vi "CRYGet Curve & Sensitiviy.vi"(9 "Calibration Cluster":T1={"Calibration"={"Calibration Step Name"="", "Device"="", "Correction Curve Name"="", "Equalization Curve Name"="", "Sensitivity Curve Name"="", "Corr Folder and File"="", "EQ Folder and File"="", "Sens Folder and File"="", "Corr Step size"=0, "EQ Step size"=0, "Input"=FALSE, "Last Cal Date (sec)"=timestamp(0 s since 1904-01-01), "Cha Name"="", "Corr Curve Found"=FALSE, "EQ Curve Found"=FALSE, "Sens Curve Found"=FALSE, "Signal Type"="", "Calibrated Device"="", "Hz"=0}, "Corr Curve"={"Name"="", "Curve"=[], "X data"=1, "Y data"=1, "Z data"=1, "X axis"=0, "Y axis"=1, "Z axis"=1, "X unit"="Hz", "Y unit"="", "Z unit"="deg.", "X dB ref"=1.0, "Y dB ref"=1.0, "Z dB ref"=1.0, "single val"=FALSE, "protected"=FALSE, "display X"=TRUE, "display Y"=TRUE, "display Z"=TRUE, "Test Info"="", "Step No."=0, "Plot Settings"={"Color"=0, "Interpolation"=0, "Point Style"=0, "Line Style"=0, "Point Color"=0, "Line Width"=0, "Bar Plot Style"=0, "Fill To"=0}, "AutoProtect"=FALSE}, "EQ Curve"={"Name"="", "Curve"=[], "X data"=1, "Y data"=1, "Z data"=1, "X axis"=0, "Y axis"=1, "Z axis"=1, "X unit"="Hz", "Y unit"="", "Z unit"="deg.", "X dB ref"=1.0, "Y dB ref"=1.0, "Z dB ref"=1.0, "single val"=FALSE, "protected"=FALSE, "display X"=TRUE, "display Y"=TRUE, "display Z"=TRUE, "Test Info"="", "Step No."=0, "Plot Settings"={"Color"=0, "Interpolation"=0, "Point Style"=0, "Line Style"=0, "Point Color"=0, "Line Width"=0, "Bar Plot Style"=0, "Fill To"=0}, "AutoProtect"=FALSE}, "Sens Curve"={"Name"="", "Curve"=[], "X data"=1, "Y data"=1, "Z data"=1, "X axis"=0, "Y axis"=1, "Z axis"=1, "X unit"="Hz", "Y unit"="", "Z unit"="deg.", "X dB ref"=1.0, "Y dB ref"=1.0, "Z dB ref"=1.0, "single val"=FALSE, "protected"=FALSE, "display X"=TRUE, "display Y"=TRUE, "display Z"=TRUE, "Test Info"="", "Step No."=0, "Plot Settings"={"Color"=0, "Interpolation"=0, "Point Style"=0, "Line Style"=0, "Point Color"=0, "Line Width"=0, "Bar Plot Style"=0, "Fill To"=0}, "AutoProtect"=FALSE}} {"Sens Curve"."Z data" items=["dB", "Lin"]; "Sens Curve"."X data" items=["dB", "Lin"]; "Sens Curve"."Y data" items=["dB", "Lin"]; "Sens Curve"."Z dB ref" format="%.1f"; "Sens Curve"."Z axis" items=["Log", "Lin"]; "Sens Curve"."X dB ref" format="%.1f"; "Sens Curve"."X axis" items=["Log", "Lin"]; "Sens Curve"."Y axis" items=["Log", "Lin"]; "Sens Curve"."Y dB ref" format="%.1f"; "Sens Curve"."Curve"."z" format="%.2f"; "Sens Curve"."Curve"."y" format="%.2f"; "Sens Curve"."Curve"."x" format="%.2f"; "EQ Curve"."Z data" items=["dB", "Lin"]; "EQ Curve"."X data" items=["dB", "Lin"]; "EQ Curve"."Y data" items=["dB", "Lin"]; "EQ Curve"."Z dB ref" format="%.1f"; "EQ Curve"."Z axis" items=["Log", "Lin"]; "EQ Curve"."X dB ref" format="%.1f"; "EQ Curve"."X axis" items=["Log", "Lin"]; "EQ Curve"."Y axis" items=["Log", "Lin"]; "EQ Curve"."Y dB ref" format="%.1f"; "EQ Curve"."Curve"."z" format="%.2f"; "EQ Curve"."Curve"."y" format="%.2f"; "EQ Curve"."Curve"."x" format="%.2f"; "Corr Curve"."Z data" items=["dB", "Lin"]; "Corr Curve"."X data" items=["dB", "Lin"]; "Corr Curve"."Y data" items=["dB", "Lin"]; "Corr Curve"."Z dB ref" format="%.1f"; "Corr Curve"."Z axis" items=["Log", "Lin"]; "Corr Curve"."X dB ref" format="%.1f"; "Corr Curve"."X axis" items=["Log", "Lin"]; "Corr Curve"."Y axis" items=["Log", "Lin"]; "Corr Curve"."Y dB ref" format="%.1f"; "Corr Curve"."Curve"."z" format="%.2f"; "Corr Curve"."Curve"."y" format="%.2f"; "Corr Curve"."Curve"."x" format="%.2f"; "Calibration"."EQ Step size" items=["R10", "R20", "R40", "R80", "User"]; "Calibration"."Corr Step size" items=["R10", "R20", "R40", "R80", "User"]}, 10 "Finished test? (T)":bool=TRUE, 11 "Data stack out":T4 {"Z data" items=["dB", "Lin"]; "X data" items=["dB", "Lin"]; "Y data" items=["dB", "Lin"]; "Z dB ref" format="%.1f"; "Z axis" items=["Log", "Lin"]; "X dB ref" format="%.1f"; "X axis" items=["Log", "Lin"]; "Y axis" items=["Log", "Lin"]; "Y dB ref" format="%.1f"; "Curve"."z" format="%.2f"; "Curve"."y" format="%.2f"; "Curve"."x" format="%.2f"}) -> (0 "Success?":bool, 1 "Sensitivity":dbl format="%.2f", 2 "corr-out curve":cluster{"x":dbl, "y":dbl, "z":dbl}[](array[cluster]) {"z" format="%.2f"; "y" format="%.2f"; "x" format="%.2f"}, 3 "eq- out curve":cluster{"x":dbl, "y":dbl, "z":dbl}[](array[cluster]) {"z" format="%.2f"; "y" format="%.2f"; "x" format="%.2f"})   [LabVIEW 2013]
uses:
  Typedef Control/CRYData Cluster Array.ctl
  Typedef Control/CRYData Cluster.ctl
  Typedef Control/CRYCalibration 2DCluster.ctl
  Typedef Control/CRYCalibration Cluster.ctl
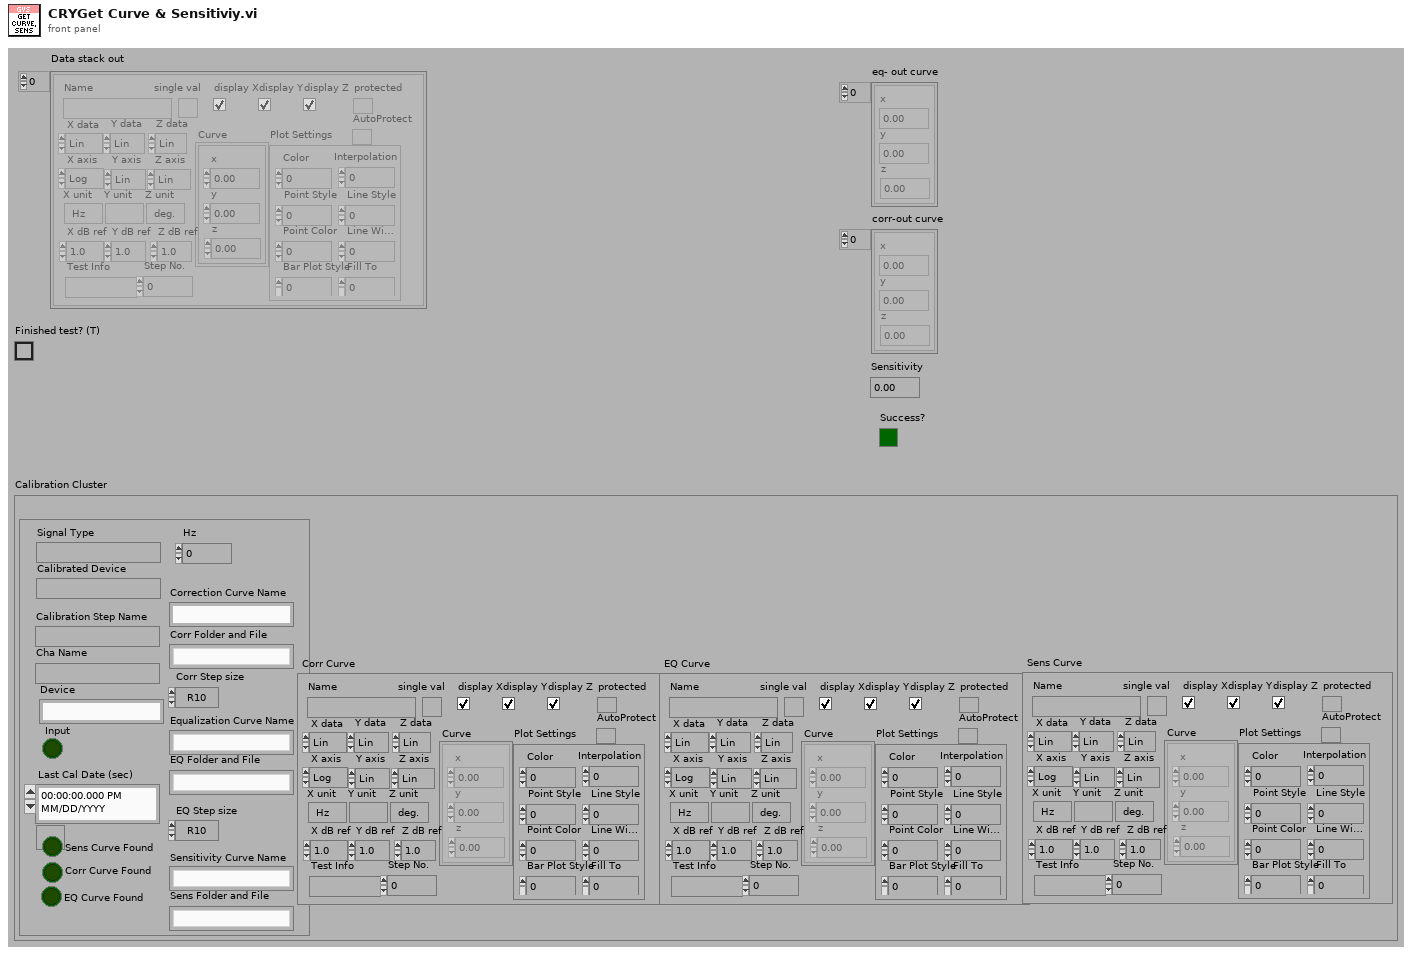
[diagram p1: front panel]
types:
  T1 = typedef "CRYCalibration 2DCluster.ctl" = cluster{"Calibration":T2, "Corr Curve":T3, "EQ Curve":T3, "Sens Curve":T3}
  T2 = typedef "CRYCalibration Cluster.ctl" = cluster{"Calibration Step Name":string, "Device":string, "Correction Curve Name":string, "Equalization Curve Name":string, "Sensitivity Curve Name":string, "Corr Folder and File":string, "EQ Folder and File":string, "Sens Folder and File":string, "Corr Step size":u16, "EQ Step size":u16, "Input":bool, "Last Cal Date (sec)":timestamp, "Cha Name":string, "Corr Curve Found":bool, "EQ Curve Found":bool, "Sens Curve Found":bool, "Signal Type":string, "Calibrated Device":string, "Hz":u32}
  T3 = typedef "CRYData Cluster.ctl" = cluster{"Name":string, "Curve":cluster{"x":dbl, "y":dbl, "z":dbl}[], "X data":u16, "Y data":u16, "Z data":u16, "X axis":u16, "Y axis":u16, "Z axis":u16, "X unit":string, "Y unit":string, "Z unit":string, "X dB ref":dbl, "Y dB ref":dbl, "Z dB ref":dbl, "single val":bool, "protected":bool, "display X":bool, "display Y":bool, "display Z":bool, "Test Info":string, "Step No.":i32, "Plot Settings":cluster{"Color":u32, "Interpolation":u8, "Point Style":u8, "Line Style":u8, "Point Color":u32, "Line Width":u8, "Bar Plot Style":u8, "Fill To":i16}, "AutoProtect":bool}
  T4 = typedef "CRYData Cluster Array.ctl" = T3[]
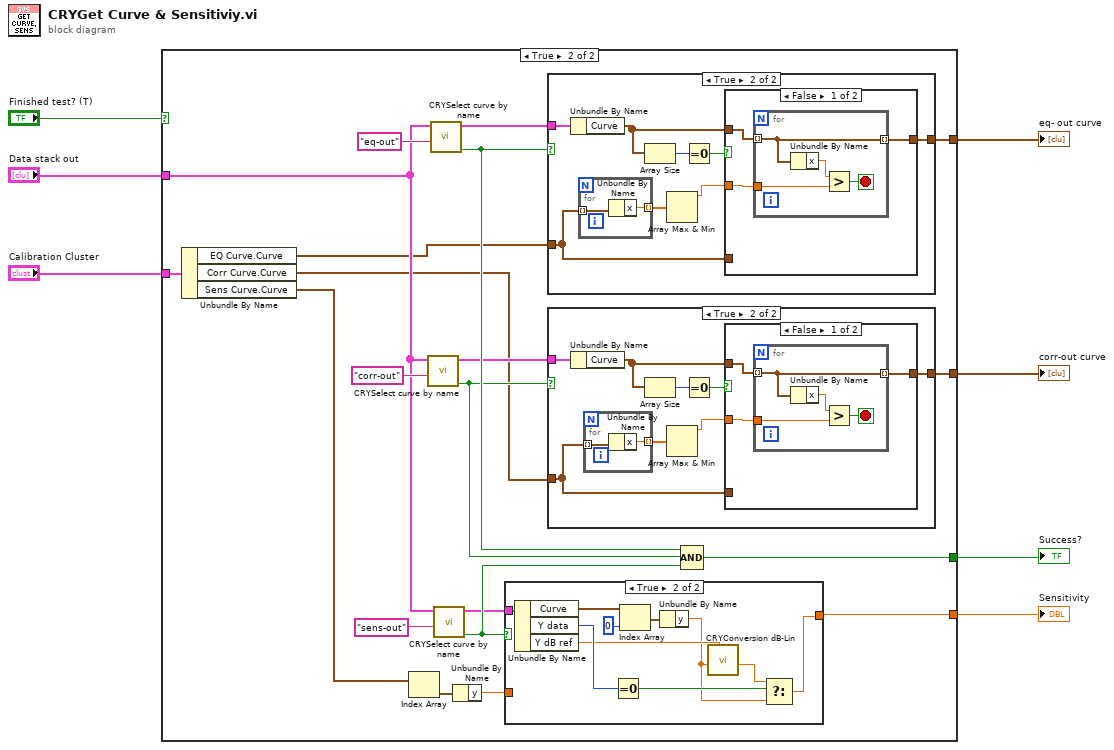
[diagram p0: block diagram]
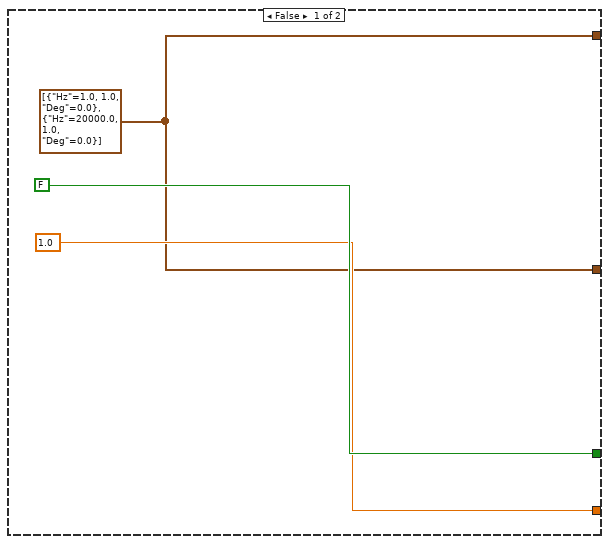
[diagram p2: hidden frame]
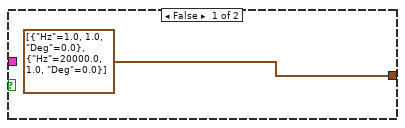
[diagram p3: hidden frame]
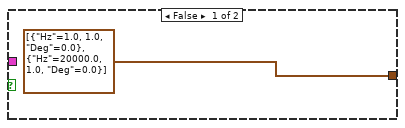
[diagram p6: hidden frame]
diagram:
  n1 = case shown="True" "Finished test? (T)" {
    tunnel: [w8 w24] -> w7
    tunnel: [FALSE w29] -> w6
    tunnel: [1.0 ("y") w28] -> w5
    tunnel: [w8 w14] -> w3
    tunnel: "Data stack out" -> [_ w20]
    tunnel: "Calibration Cluster" -> [_ w19]
    frame False {
      w8 = cluster{"Hz":dbl, dbl, "Deg":dbl}[] [{"Hz"=1.0, 1.0, "Deg"=0.0}, {"Hz"=20000.0, 1.0, "Deg"=0.0}] ("Correction In")
    }
    frame True {
      n2 = Unbundle By Name(w19) -> ("EQ Curve.Curve"=w18:cluster{"x":dbl, "y":dbl, "z":dbl}[], "Corr Curve.Curve"=w15:cluster{"x":dbl, "y":dbl, "z":dbl}[], "Sens Curve.Curve"=w13:cluster{"x":dbl, "y":dbl, "z":dbl}[])
      n3 = Index Array(array=w13) -> (element=w12:cluster{"x":dbl, "y":dbl, "z":dbl})  [unwired: 1 in]
      n4 = call "CRYSelect curve by name.vi"("Curve name desired (just name, if flat data not wired)"="corr-out", "Data array"=w20) -> ("Exists?"=w16:bool, "Desired Curve"=w17:T3)  [unwired: 1 in, 7 out]
      n5 = call "CRYSelect curve by name.vi"("Curve name desired (just name, if flat data not wired)"="eq-out", "Data array"=w20) -> ("Exists?"=w21:bool, "Desired Curve"=w25:T3)  [unwired: 1 in, 7 out]
      n6 = call "CRYSelect curve by name.vi"("Curve name desired (just name, if flat data not wired)"="sens-out", "Data array"=w20) -> ("Exists?"=w30:bool, "Desired Curve"=w23:T3)  [unwired: 1 in, 7 out]
      n7 = Unbundle By Name(w12) -> ("y"=w11:dbl)
      n8 = case shown="True" w30 {
        tunnel: w23 -> [_ w60]
        tunnel: [w50 w51] -> w28
        tunnel: w11 -> [w50 _]
        frame False {
        }
        frame True {
          n9 = Unbundle By Name(w60) -> ("Curve"=w59:cluster{"x":dbl, "y":dbl, "z":dbl}[], "Y data"=w56:u16, "Y dB ref"=w55:dbl)
          n10 = Equal To 0?(x=w56) -> (x = 0?=w54:bool)
          n11 = Index Array(array=w59, index=0 ("Index")) -> (element=w57:cluster{"x":dbl, "y":dbl, "z":dbl})
          n12 = Unbundle By Name(w57) -> ("y"=w52:dbl)
          n13 = call "CRYConversion dB-Lin.vi"("dB ref."=w55, "Log In"=w52) -> ("Lin Out"=w53:dbl)  [unwired: 4 in, 3 out]
          n14 = Select(t=w53, s=w54, f=w52) -> (s? t:f=w51:dbl)
        }
      }
      n15 = case shown="True" w21 {
        tunnel: w25 -> [_ w69]
        tunnel: [cluster{"Hz":dbl, dbl, "Deg":dbl}[] [{"Hz"=1.0, 1.0, "Deg"=0.0}, {"Hz"=20000.0, 1.0, "Deg"=0.0}] ("Correction In") w66] -> w24
        tunnel: w18 -> [_ w62]
        frame False {
        }
        frame True {
          n16 = Unbundle By Name(w69) -> ("Curve"=w65:cluster{"x":dbl, "y":dbl, "z":dbl}[])
          n17 = for {
            tunnel: w62 -> [w79] mode=indexing
            tunnel: [w78] -> w68 mode=indexing
            n18 = Unbundle By Name(w79) -> ("x"=w78:dbl)
          }
          n19 = Array Size(array=w65) -> (size(s)=w64:i32)
          n20 = Array Max & Min(array=w68) -> (max value=w67:dbl)  [unwired: 3 out]
          n21 = Equal To 0?(x=w64) -> (x = 0?=w63:bool)
          n22 = case shown="False" w63 {
            tunnel: w67 -> [w72 _]
            tunnel: [w71 w77] -> w66
            tunnel: w65 -> [w70 _]
            tunnel: w62 -> [_ w77]
            frame False {
              n23 = for {
                tunnel: w72 -> [w75]
                tunnel: w70 -> [w73] mode=indexing
                tunnel: [w73] -> w71 mode=indexing
                stop <- w74 stop-if-true
                n24 = Unbundle By Name(w73) -> ("x"=w76:dbl)
                n25 = Greater?(x=w76, y=w75) -> (0:w74:bool)
              }
            }
            frame True {
            }
          }
        }
      }
      n26 = case shown="True" w16 {
        tunnel: w17 -> [_ w39]
        tunnel: [cluster{"Hz":dbl, dbl, "Deg":dbl}[] [{"Hz"=1.0, 1.0, "Deg"=0.0}, {"Hz"=20000.0, 1.0, "Deg"=0.0}] ("Correction In") w36] -> w14
        tunnel: w15 -> [_ w32]
        frame False {
        }
        frame True {
          n27 = Unbundle By Name(w39) -> ("Curve"=w35:cluster{"x":dbl, "y":dbl, "z":dbl}[])
          n28 = for {
            tunnel: w32 -> [w49] mode=indexing
            tunnel: [w48] -> w38 mode=indexing
            n29 = Unbundle By Name(w49) -> ("x"=w48:dbl)
          }
          n30 = Array Size(array=w35) -> (size(s)=w34:i32)
          n31 = Array Max & Min(array=w38) -> (max value=w37:dbl)  [unwired: 3 out]
          n32 = Equal To 0?(x=w34) -> (x = 0?=w33:bool)
          n33 = case shown="False" w33 {
            tunnel: w37 -> [w42 _]
            tunnel: [w41 w47] -> w36
            tunnel: w35 -> [w40 _]
            tunnel: w32 -> [_ w47]
            frame False {
              n34 = for {
                tunnel: w42 -> [w45]
                tunnel: w40 -> [w43] mode=indexing
                tunnel: [w43] -> w41 mode=indexing
                stop <- w44 stop-if-true
                n35 = Unbundle By Name(w43) -> ("x"=w46:dbl)
                n36 = Greater?(x=w46, y=w45) -> (0:w44:bool)
              }
            }
            frame True {
            }
          }
        }
      }
      n37 = Compound Arithmetic op=AND(w21, w16, w30) -> (w29:bool)
    }
  }
  "corr-out curve" <- w3
  "Sensitivity" <- w5
  "eq- out curve" <- w7
  "Success?" <- w6
